vi "Drive_Cmd_Cheesey_Drive.vi"(6 "Sens Values":T1={"Quickturn_Sens_High"=1.0, "Quickturn_Sens_Low"=1.0}, 8 "gear shift state":enum16{"low", "high"}(ring), 9 "Wheel":dbl, 10 "Throttle":dbl, 11 "Drive Loop Cluster":T2={"Sensor Data"={"Gyro Data"={"Gyro RT FIFO"=refnum, "Gyro Current"=0.0, "Gyro Hold"=0.0}, "Encoder Data"={"Encoder RT FIFO"=refnum, "Encoder Current"=0.0, "Encoder Hold"=0.0}, "Camera Data"={"Camera RT FIFO"=refnum, "Camera Current"={" Angle"=0.0, "Valid"=FALSE}}}, "PID Update"=refnum, "RobotDriveDevRef"={"DevStatus"={"status"=FALSE, "code"=0, "source"=""}, "Motors[]"=[], "Square Inputs"=FALSE, "Max Output"=1.0}, "Drive Train"=enum."Tank Drive 2 Motor", "Valid Commands"=[], "Drive Comand Notifier"=refnum}) -> ()   [LabVIEW 2016]
doc: "Help writen by FRC Team 836 - The RoboBees\n\nVI places robot in manual drive mode with speed and steering commands.\n\nThis VI takes throttle and steering commands and writes them with the \"Manual\" mode command to the Drive Command RT FIFO in the\nDrive Loop Cluster.\n\nThe RT FIFO has to be initialized using the \"Drive_Loop_Initialize_w_Help\" VI."
uses:
  <userlib>/836-Library/Drive/Drive_Code_V2/Drive_Code_Support/Drive_Code_Bundle.ctl
  <userlib>/836-Library/Drive/Drive_Code_V2/Drive_Code_Support/SensorTypedefs/Sensor_Cluster.ctl
  <userlib>/836-Library/Drive/Drive_Code_V2/Drive_Code_Support/SensorTypedefs/Camera_Cluster.ctl
  <userlib>/836-Library/Drive/Drive_Code_V2/Drive_Code_Support/Drive_Code_PID_Bundle.ctl
  <vilib>/Rock Robotics/WPI/RobotDrive/WPI_RobotDriveDevRef.ctl
  <vilib>/Rock Robotics/WPI/MotorControl/WPI_MotorControlDeviceRef.ctl
  <vilib>/Rock Robotics/WPI/MotorControl/WPI_MotorControlType.ctl
  <vilib>/Rock Robotics/SystemInterfaces/DIO/FPGA_DIOPWMChannel.ctl
  <vilib>/Rock Robotics/WPI/PWM/WPI_PWMDeadband.ctl
  <userlib>/836-Library/Drive/Drive_Code_V2/Drive_Code_Support/DriveTrains/Drive_Trains.ctl
  <userlib>/836-Library/Drive/Drive_Code_V2/Drive_Code_Support/Command_Sends/Drive_Code_Command_Type.ctl
  <userlib>/836-Library/Drive/Drive_Code_V2/Drive_Code_Support/Command_Sends/Drive_Code_Command_List.ctl
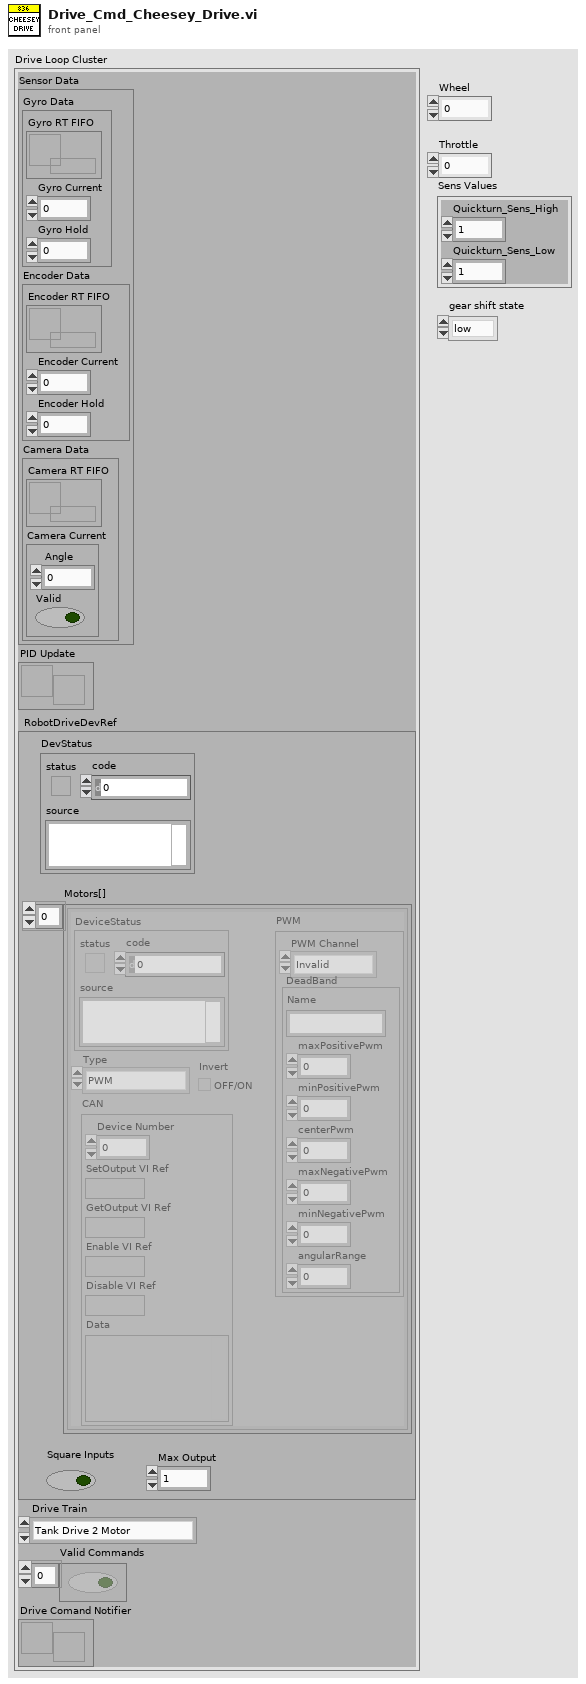
[diagram p1: front panel]
types:
  T1 = cluster{"Quickturn_Sens_High":dbl, "Quickturn_Sens_Low":dbl}
  T2 = typedef "Drive_Code_Bundle.ctl" = cluster{"Sensor Data":T3, "PID Update":refnum<notifier>, "RobotDriveDevRef":T5, "Drive Train":T10, "Valid Commands":bool[], "Drive Comand Notifier":refnum<notifier>}
  T3 = typedef "Sensor_Cluster.ctl" = cluster{"Gyro Data":cluster{"Gyro RT FIFO":refnum<k33>, "Gyro Current":dbl, "Gyro Hold":dbl}, "Encoder Data":cluster{"Encoder RT FIFO":refnum<k33>, "Encoder Current":dbl, "Encoder Hold":dbl}, "Camera Data":cluster{"Camera RT FIFO":refnum<k33>, "Camera Current":T4}}
  T4 = typedef "Camera_Cluster.ctl" = cluster{" Angle":dbl, "Valid":bool}
  T5 = typedef "WPI_RobotDriveDevRef.ctl" = cluster{"DevStatus":errorcluster, "Motors[]":T6[], "Square Inputs":bool, "Max Output":dbl}
  T6 = typedef "WPI_MotorControlDeviceRef.ctl" = cluster{"DeviceStatus":errorcluster, "Type":T7, "PWM":cluster{"PWM Channel":T8, "DeadBand":T9}, "CAN":cluster{"Device Number":u8, "SetOutput VI Ref":variant, "GetOutput VI Ref":variant, "Enable VI Ref":variant, "Disable VI Ref":variant, "Data":variant}, "Invert":bool}
  T7 = typedef "WPI_MotorControlType.ctl" = enum16{"PWM", "CAN"}
  T8 = typedef "FPGA_DIOPWMChannel.ctl" = enum8{"PWM 0", "PWM 1", "PWM 2", "PWM 3", "PWM 4", "PWM 5", "PWM 6", "PWM 7", "PWM 8", "PWM 9", "PWM MXP 0", "PWM MXP 1", "PWM MXP 2", "PWM MXP 3", "PWM MXP 4", "PWM MXP 5", "PWM MXP 6", "PWM MXP 7", "PWM MXP 8", "PWM MXP 9", "Invalid"}
  T9 = typedef "WPI_PWMDeadband.ctl" = cluster{"Name":string, "maxPositivePwm":i32, "minPositivePwm":i32, "centerPwm":i32, "maxNegativePwm":i32, "minNegativePwm":i32, "angularRange":u16}
  T10 = typedef "Drive_Trains.ctl" = enum16{"Tank Drive 2 Motor", "Tank Drive 4 Motor", "Mecanum Drive", "Kiwi Drive"}
  T11 = typedef "Drive_Code_Command_List.ctl" = enum16{"Do Nothing", "Manual", "Drive Continuous", "Turn", "Drive Distance", "Hold Position", "Hold Yaw", "Follow Camera", "Turn to Camera", "Approach Camera"}
  T12 = typedef "Drive_Code_Command_Type.ctl" = cluster{"Command":T11, "Parameter A":dbl, "Parameter B":dbl, "Parameter C":dbl, "Absolute?":bool}
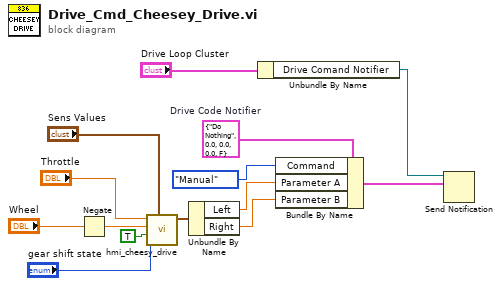
[diagram p0: block diagram]
diagram:
  w3 = T12 {"Command"=enum."Do Nothing", "Parameter A"=0.0, "Parameter B"=0.0, "Parameter C"=0.0, "Absolute?"=FALSE}  # Drive Code Notifier
  n1 = Negate(x="Wheel") -> (-x=w8:dbl)
  n2 = call <userlib>:"hmi_cheesy_drive.vi"("Sens Values"="Sens Values", "gear shift state"="gear shift state", "Quick Turn"=TRUE, "Wheel"=w8, "Throttle"="Throttle") -> ("Drive Data"=w9:cluster{"Left":dbl, "Right":dbl})  [unwired: 6 in]
  n3 = Unbundle By Name(w9) -> ("Left"=w10:dbl, "Right"=w11:dbl)
  n4 = Unbundle By Name("Drive Loop Cluster") -> ("Drive Comand Notifier"=w14:refnum<notifier>)
  n5 = Bundle By Name(cluster=w3, "Command"=Drive_Code_Command_List."Manual", "Parameter A"=w10, "Parameter B"=w11) -> (w13:T12)
  n6 = Send Notification(notification=w13, notifier=w14) -> ()  [unwired: 1 in, 2 out]
